vi "GetText.vi"(8 "error in":errorcluster, 11 "TDMS datalogger editor node in":refnum<class "TDMS datalogger editor node.lvclass">) -> (0 "error out":errorcluster, 1 "additional text":string, 2 "text":string, 3 "TDMS datalogger editor node out":refnum<class "TDMS datalogger editor node.lvclass">, 4 "glyph":string)   [LabVIEW 2013, in "TDMS datalogger editor node.lvclass"]
uses:
  TDMS datalogger editor node.lvclass
  <vilib>/NI/Tag Bus Data Framework/Configuration Editor/Classes/Module editor node/module editor node.lvclass
  <vilib>/NI/Tag Bus Data Framework/Configuration Editor/PL Framework Configuration Tool.lvlib
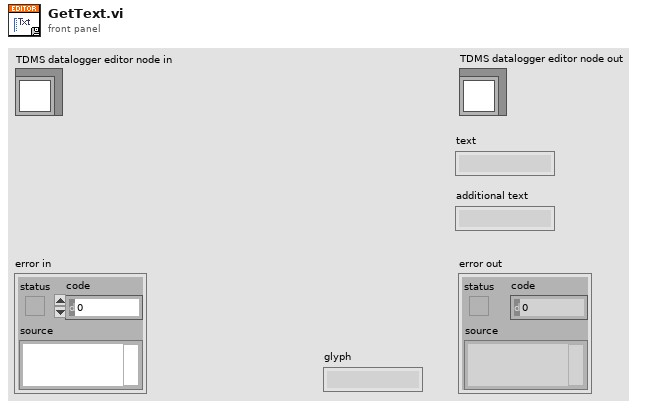
[diagram p1: front panel]
types:
  T1 = typedef "PL Framework Configuration Tool.lvlib/Glyphs Status.ctl" = enum16{"Normal", "Error"}
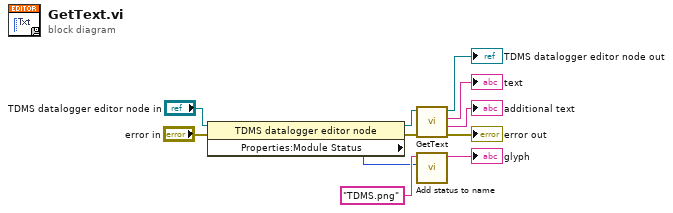
[diagram p0: block diagram]
diagram:
  n1 = property class="TDMS datalogger editor node"(reference="TDMS datalogger editor node in", error in="error in") -> (reference out=w4:refnum<class "TDMS datalogger editor node.lvclass">, error out=w6:errorcluster, "Properties:Module Status"=w10:T1)
  n2 = call-parent "GetText.vi"("error in"=w6, "Module Editor Node in"=w4) -> ("error out"=→"error out":errorcluster, "additional text"=→"additional text":string, "text"=→"text":string, "Module Editor Node out"=→"TDMS datalogger editor node out":refnum<class "TDMS datalogger editor node.lvclass">)  [unwired: 5 in, 1 out]
  n3 = call <vilib>:"Add status to name.vi"("Status"=w10, "Name"="TDMS.png" ("glyph")) -> ("Name with status"=→"glyph":string)  [unwired: 9 in]
